vi "手动启动选择对话框.vi"() -> (2 "确定":bool, 3 "参数启用":T1)   [LabVIEW 2016, in "PLC.lvlib"]
uses:
  PLC.lvlib
panel:
  in  "总氮":bool
  in  "CODCr":bool
  in  "总磷":bool
  in  "氨氮":bool
  in  "CODmn":bool
  in  "多参数":bool
  in  "取消":bool
  in  "确定":bool
  # "请选择启动参数"
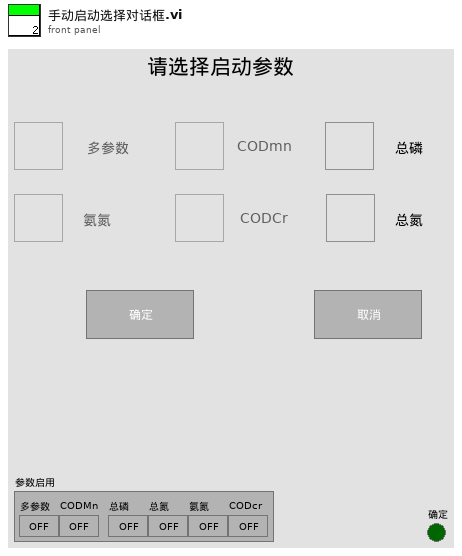
[diagram p1: front panel]
types:
  T1 = cluster{"多参数":bool, "CODMn":bool, "总磷":bool, "总氮":bool, "氨氮":bool, "CODcr":bool}
  T2 = enum8{"Enabled", "Disabled", "Disabled and Grayed Out"}
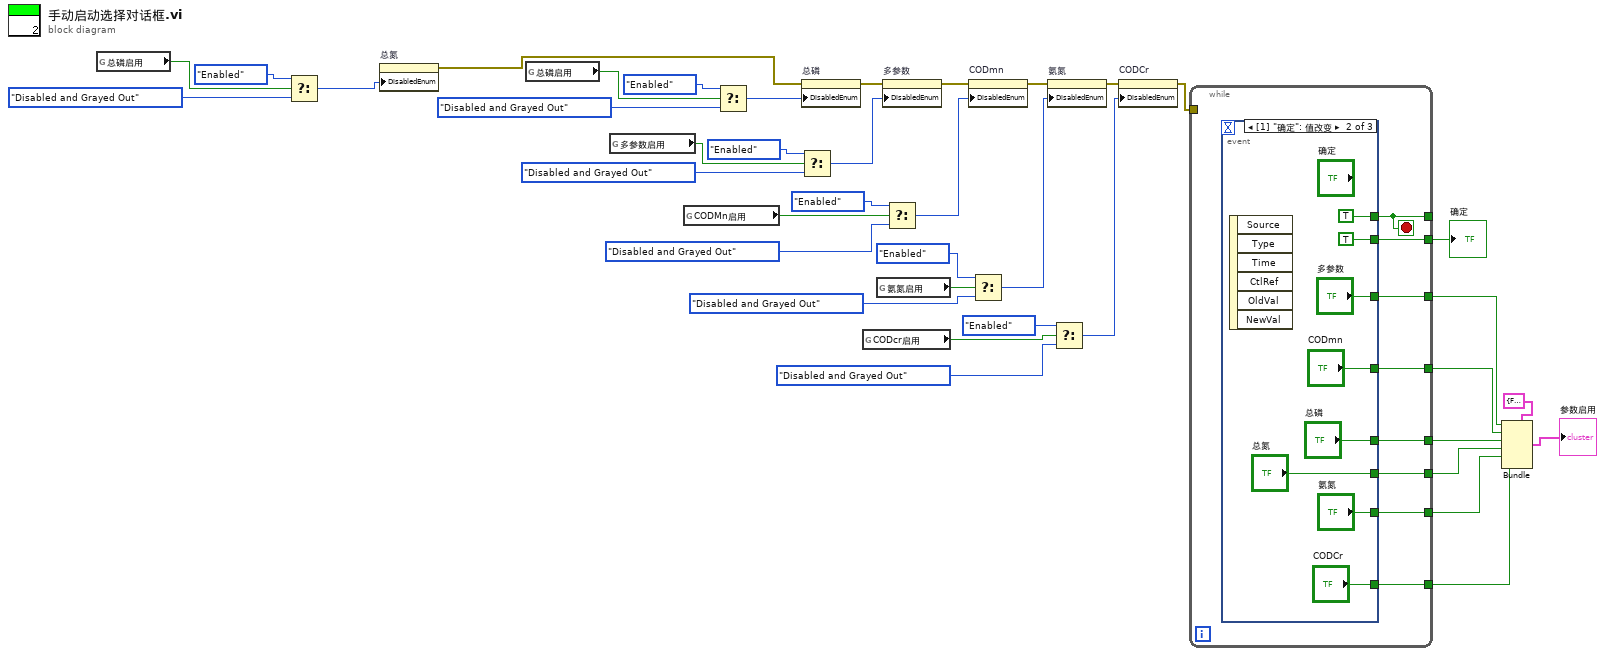
[diagram p0: block diagram]
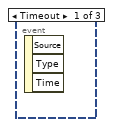
[diagram p2: hidden frame]
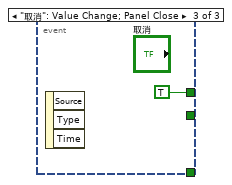
[diagram p3: hidden frame]
diagram:
  n1 = global read "系统设置全局变量.vi" "总磷启用"() -> (w9:bool)
  n2 = Select(t=T2."Enabled" ("禁用"), s=w9, f=T2."Disabled and Grayed Out" ("禁用")) -> (s? t:f=w8:T2)
  n3 = property on="总氮" class="Bool (严格)"("DisabledEnum"=w8) -> (error out=w7:errorcluster)  [unwired: 2 in, 1 out]
  n4 = global read "系统设置全局变量.vi" "总磷启用"() -> (w36:bool)
  n5 = global read "系统设置全局变量.vi" "多参数启用"() -> (w18:bool)
  n6 = global read "系统设置全局变量.vi" "CODMn启用"() -> (w22:bool)
  n7 = Select(t=T2."Enabled" ("禁用"), s=w36, f=T2."Disabled and Grayed Out" ("禁用")) -> (s? t:f=w33:T2)
  n8 = property on="总磷" class="Bool (严格)"(error in=w7, "DisabledEnum"=w33) -> (error out=w16:errorcluster)  [unwired: 1 in, 1 out]
  n9 = Select(t=T2."Enabled" ("禁用"), s=w18, f=T2."Disabled and Grayed Out" ("禁用")) -> (s? t:f=w17:T2)
  n10 = global read "系统设置全局变量.vi" "CODcr启用"() -> (w20:bool)
  n11 = global read "系统设置全局变量.vi" "氨氮启用"() -> (w24:bool)
  n12 = property on="多参数" class="Bool (严格)"(error in=w16, "DisabledEnum"=w17) -> (error out=w15:errorcluster)  [unwired: 1 in, 1 out]
  n13 = Select(t=T2."Enabled" ("禁用"), s=w22, f=T2."Disabled and Grayed Out" ("禁用")) -> (s? t:f=w21:T2)
  n14 = property on="CODmn" class="Bool (严格)"(error in=w15, "DisabledEnum"=w21) -> (error out=w14:errorcluster)  [unwired: 1 in, 1 out]
  n15 = Select(t=T2."Enabled" ("禁用"), s=w24, f=T2."Disabled and Grayed Out" ("禁用")) -> (s? t:f=w23:T2)
  n16 = property on="氨氮" class="Bool (严格)"(error in=w14, "DisabledEnum"=w23) -> (error out=w13:errorcluster)  [unwired: 1 in, 1 out]
  n17 = Select(t=T2."Enabled" ("禁用"), s=w20, f=T2."Disabled and Grayed Out" ("禁用")) -> (s? t:f=w19:T2)
  n18 = property on="CODCr" class="Bool (严格)"(error in=w13, "DisabledEnum"=w19) -> (error out=w12:errorcluster)  [unwired: 1 in, 1 out]
  n19 = while {
    tunnel: [w47] -> w39
    tunnel: [w46] -> w2
    tunnel: [w45] -> w37
    tunnel: [w44] -> _
    tunnel: [w43] -> w38
    tunnel: [w42] -> w4
    tunnel: [w41] -> w1
    tunnel: w12 -> [_]
    tunnel: [w40] -> w3
    stop <- w44 stop-if-true
    n20 = event shown="[1] \"确定\": 值改变" {
      selector: _ -> [_ _ _]
      dyn-events: _ -> [_ _ _]
      timeout: _ -> [_ _ _]
      tunnel: [_ TRUE TRUE] -> w44
      tunnel: [_ "多参数" _] -> w47
      tunnel: [_ "氨氮" _] -> w46
      tunnel: [_ "CODmn" _] -> w45
      tunnel: [_ TRUE _] -> w43
      tunnel: [_ "总磷" _] -> w42
      tunnel: [_ "CODCr" _] -> w41
      tunnel: [_ "总氮" _] -> w40
      event Timeout {
        n21 = event-data() -> ()  [unwired: 1 in, 3 out]
      }
      event "确定": Value Change {
        n22 = event-data() -> ()  [unwired: 1 in, 6 out]
      }
      event "取消": Value Change; Panel Close {
        n23 = event-data() -> ()  [unwired: 1 in, 3 out]
      }
    }
  }
  "确定" <- w38
  n24 = Bundle(cluster=T1 {"多参数"=FALSE, "CODMn"=FALSE, "总磷"=FALSE, "总氮"=FALSE, "氨氮"=FALSE, "CODcr"=FALSE} ("参数启用"), "多参数"=w39, "CODMn"=w37, "总磷"=w4, "总氮"=w3, "氨氮"=w2, "CODcr"=w1) -> (→"参数启用":T1)
